vi "Clic.vi"(5 "Amplitude (V)":dbl=1.0 max=19.0 step=1.0, 6 "Stimulation freq (stim/sec)":u32=20, 7 "Fs (#S/s)":dbl=200000.0) -> (0 "Stimulus Waveform":waveform(dbl)(graph), 1 "Stimulus duration (ms)":dbl=0.035, 2 "Delay (ms)":dbl=1.0, 3 "Signal duration (#S)":dbl, 4 "Signal duration (ms)":dbl)   [LabVIEW 2014]
uses:
  <vilib>/Analysis/NI_AALBase.lvlib
panel:
  in  "Clic duration (ms)":dbl=0.035
  out "Clic duration (#S)":dbl
  out "Amplitude (1/10 V)":dbl
  out "Delay (#S)":dbl
  # "Stimulus Configuration"
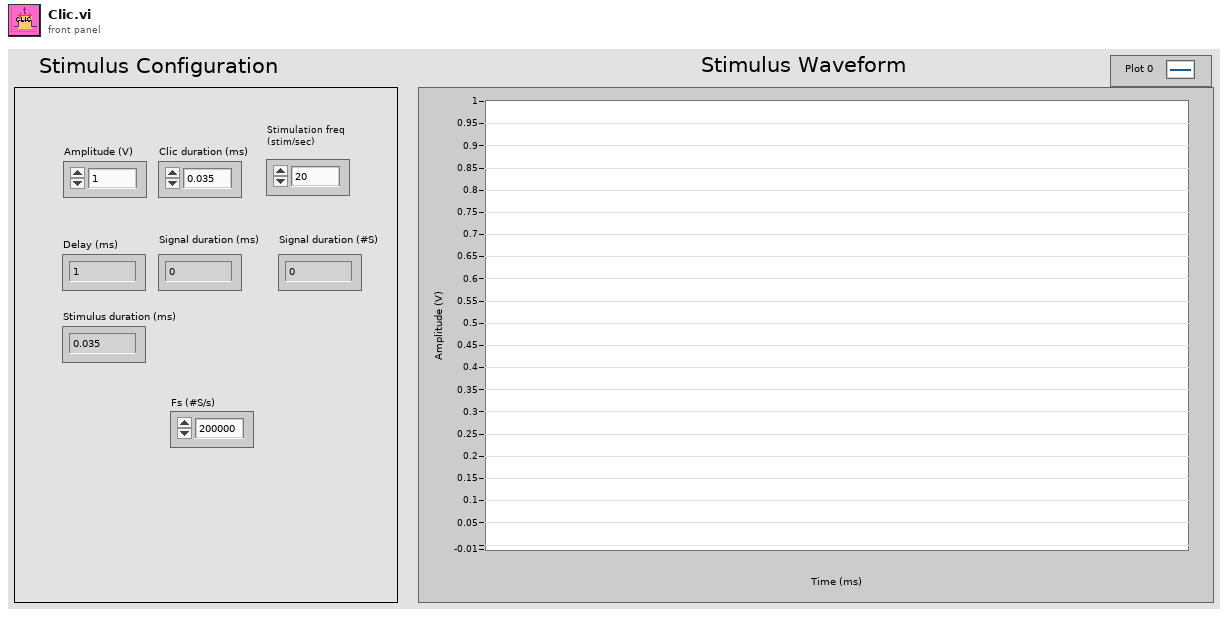
[diagram p1: front panel]
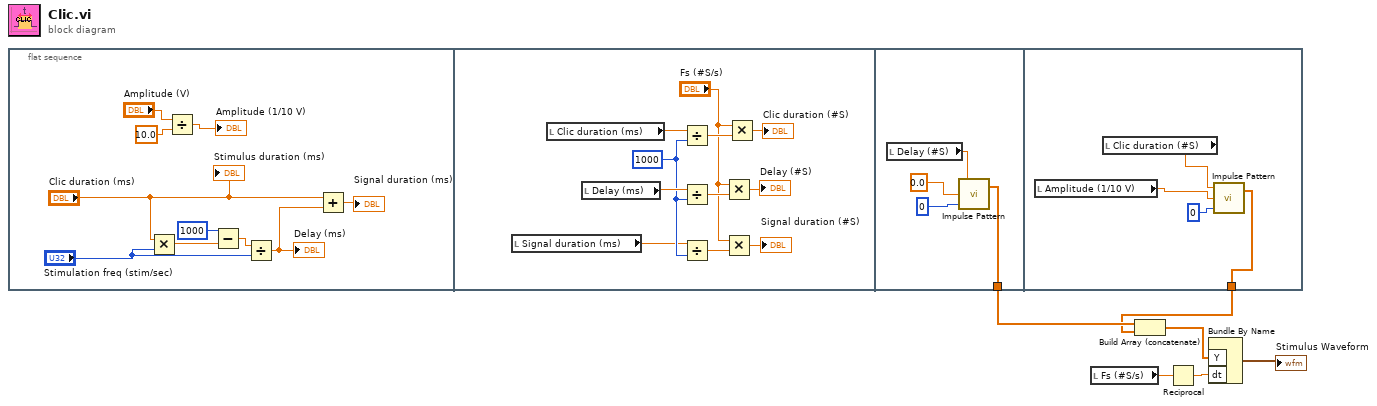
[diagram p0: block diagram]
diagram:
  n1 = flat-sequence {
    tunnel: [w28] -> w3
    tunnel: [w35] -> w2
    frame #0 {
      n2 = Multiply(x="Clic duration (ms)", y="Stimulation freq (stim/sec)") -> (x*y=w13:dbl)
      n3 = Divide(x="Amplitude (V)", y=10.0) -> (x/y=→"Amplitude (1/10 V)":dbl)
      n4 = Subtract(x=1000, y=w13) -> (x-y=w10:dbl)
      n5 = Divide(x=w10, y="Stimulation freq (stim/sec)") -> (x/y=w8:dbl)
      "Delay (ms)" <- w8
      n6 = Add(x="Clic duration (ms)", y=w8) -> (x+y=→"Signal duration (ms)":dbl)
      "Stimulus duration (ms)" <- "Clic duration (ms)"
    }
    frame #1 {
      w18 = 1000
      n7 = local read "Signal duration (ms)"() -> (w17:dbl)
      n8 = local read "Clic duration (ms)"() -> (w27:dbl)
      n9 = local read "Delay (ms)"() -> (w24:dbl)
      n10 = Divide(x=w27, y=w18) -> (x/y=w26:dbl)
      n11 = Divide(x=w24, y=w18) -> (x/y=w22:dbl)
      n12 = Divide(x=w17, y=w18) -> (x/y=w21:dbl)
      n13 = Multiply(x="Fs (#S/s)", y=w22) -> (x*y=→"Delay (#S)":dbl)
      n14 = Multiply(x="Fs (#S/s)", y=w21) -> (x*y=→"Signal duration (#S)":dbl)
      n15 = Multiply(x="Fs (#S/s)", y=w26) -> (x*y=→"Clic duration (#S)":dbl)
    }
    frame #2 {
      n16 = local read "Delay (#S)"() -> (w31:dbl)
      n17 = call <vilib>:"Impulse Pattern.vi"("delay"=0, "amplitude"=0.0, "samples"=w31) -> ("Impulse Pattern"=w28:dbl[])  [unwired: 1 out]
    }
    frame #3 {
      n18 = local read "Amplitude (1/10 V)"() -> (w33:dbl)
      n19 = local read "Clic duration (#S)"() -> (w32:dbl)
      n20 = call <vilib>:"Impulse Pattern.vi"("delay"=0, "amplitude"=w33, "samples"=w32) -> ("Impulse Pattern"=w35:dbl[])  [unwired: 1 out]
    }
  }
  n21 = local read "Fs (#S/s)"() -> (w6:dbl)
  n22 = Build Array (concatenate)(w3, w2) -> (w4:dbl[])
  n23 = Reciprocal(x=w6) -> (1/x=w5:dbl)
  n24 = Bundle By Name("Y"=w4, "dt"=w5) -> (→"Stimulus Waveform":waveform(dbl))  [unwired: 1 in]
